vi "Teleop.vi"(10 "Match Info":T2={"Autonomous Elapsed Seconds"=0.0, "TeleOp Elapsed Seconds"=1423.678, "Disabled Elapsed Seconds"=30.39, "Visited Autonomous"=FALSE, "Visited TeleOp"=TRUE, "Visited Disabled"=TRUE, "Autonomous Settings"={"Autonomous Style"=enum."Independent", "VI Refnum"=refnum}}, 11 "Call Context":T3=enum."Execute") -> ()   [LabVIEW 2012]
doc: "This VI is called for each TeleOp packet received from the DS where the robot is not disabled. It is often used to read from the joysticks and update I/O or to update setpoints for timed control loops. It should complete and return within 20 milliseconds or it may miss DS packets."
uses:
  <vilib>/Rock Robotics/WPI/DriverStation/WPI_DriverStationDerivedRobotMode.ctl
  <vilib>/Rock Robotics/WPI/DriverStation/WPI_DriverStationMatch Info.ctl
  Driver/ADXL345 I2C Axis.ctl
  Robot Global Data.vi
  <vilib>/Rock Robotics/WPI/Solenoid/Deprecated/WPI_SolenoidSetBool.vi
  <vilib>/Rock Robotics/WPI/Joystick/WPI_JoystickGetSetRefNum.vi
panel:
  in  "Speed\nLoop Gain":dbl=1.5 step=0.1
  out "Speed feet/sec":dbl[](array[numeric])=[3.755830108947835e-15, 1.6772788571212362e-15] format="%#_4f"
  in  "Right Motor Speed":dbl(slide)=0.20408163265306145 scale=-10.0..10.0
  in  "Reset Gyro":bool
  in  "Reset Distance":bool
  out "Gyro\nAngle":dbl=356.1354393216929
  in  "SLGain\nOLD ROBOT":dbl=4.000000000000003 step=0.1
  out "Loop Time":dbl=0.023
  in  "Enable Speed Control":bool=TRUE
  out "Motor Chart":T1(graph)={"Right Motor Output"=-0.0009300018600037199, "Speed"=3.755830108947835e-15, "Speed"=1.6772788571212362e-15}
  out "Distance":dbl[](array[numeric])=[109.47032085561497, 100.94278074866311] format="%#_4f"
  out "Accelerometer Chart":cluster{"Output":dbl, dbl}(graph)={"Output"=-1.6895785716878318, -1.90123646461443}
  in  "Pitch avg.#":dbl=0.95
  out "Pitch Angle":dbl(knob)=-1.6895785716878318 scale=20.0..-20.0 scale format="%#_3g"
  in  "Left Motor Speed":dbl(slide)=0.4081632653061227 scale=-10.0..10.0
  in  "Enable Auto-Balance":bool
  out "Wheel Angles":dbl[](array[knob])=[15.270320855614973, 6.742780748663112] scale=0.0..18.84
  # "Speed Loop"
  # "1.5"
  # "4.0 on 2011 robot"
  # "2.5 on home unit"
  # "FOR TESTING ONLY"
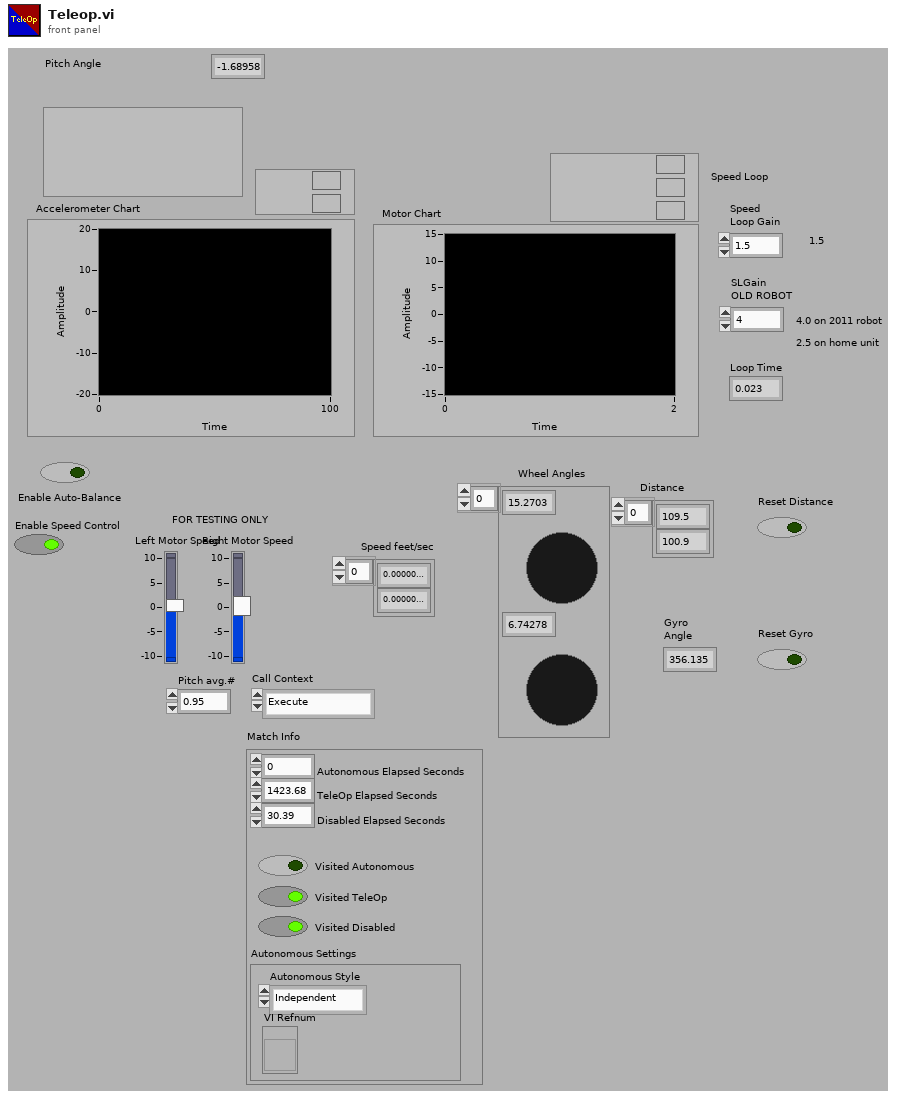
[diagram p1: front panel]
types:
  T1 = cluster{"Right Motor Output":dbl, "Speed":dbl, "Speed":dbl}
  T2 = typedef "WPI_DriverStationMatch Info.ctl" = cluster{"Autonomous Elapsed Seconds":dbl, "TeleOp Elapsed Seconds":dbl, "Disabled Elapsed Seconds":dbl, "Visited Autonomous":bool, "Visited TeleOp":bool, "Visited Disabled":bool, "Autonomous Settings":cluster{"Autonomous Style":enum16{"Iterative", "Independent"}, "VI Refnum":refnum<vi>}}
  T3 = typedef "WPI_DriverStationDerivedRobotMode.ctl" = enum16{"Init", "Execute", "Stop"}
  T4 = typedef "ADXL345 I2C Axis.ctl" = u8
  T5 = typedef "WPI_JoystickDevRef.ctl" = cluster{"Device":T6}
  T6 = typedef "WPI_JoystickDeviceEnum.ctl" = enum16{"USB 1", "USB 2", "USB 3", "USB 4", "Kinect 1", "Kinect 2"}
  T7 = typedef "WPI_JoystickButtonState.ctl" = cluster{"Button 1":bool, "Button 2":bool, "Button 3":bool, "Button 4":bool, "Button 5":bool, "Button 6":bool, "Button 7":bool, "Button 8":bool, "Button 9":bool, "Button 10":bool, "Button 11":bool, "Button 12":bool}
  T8 = typedef "WPI_SolenoidDevRef.ctl" = cluster{"DevStatus":errorcluster, "Solenoid Module":T9, "Forward Solenoid Channel":T10, "Reverse Solenoid Channel":T10}
  T9 = typedef "FPGA_TypedefSolenoidModule.ctl" = enum16{"Solenoid Module 1", "Solenoid Module 2"}
  T10 = typedef "WPI_SolenoidChannel.ctl" = enum8{"Solenoid 1", "Solenoid 2", "Solenoid 3", "Solenoid 4", "Solenoid 5", "Solenoid 6", "Solenoid 7", "Solenoid 8", "Invalid"}
  T11 = typedef "WPI_I2CDevRef.ctl" = cluster{"DevStatus":errorcluster, "Digital Module":T12, "Device Address":u8}
  T12 = typedef "FPGA_TypedefDigitalModule.ctl" = enum16{"Digital Module 1", "Digital Module 2"}
  T13 = cluster{"Left Motor Out":dbl, "Current angle (deg)":dbl, "Current angle (deg)":dbl}
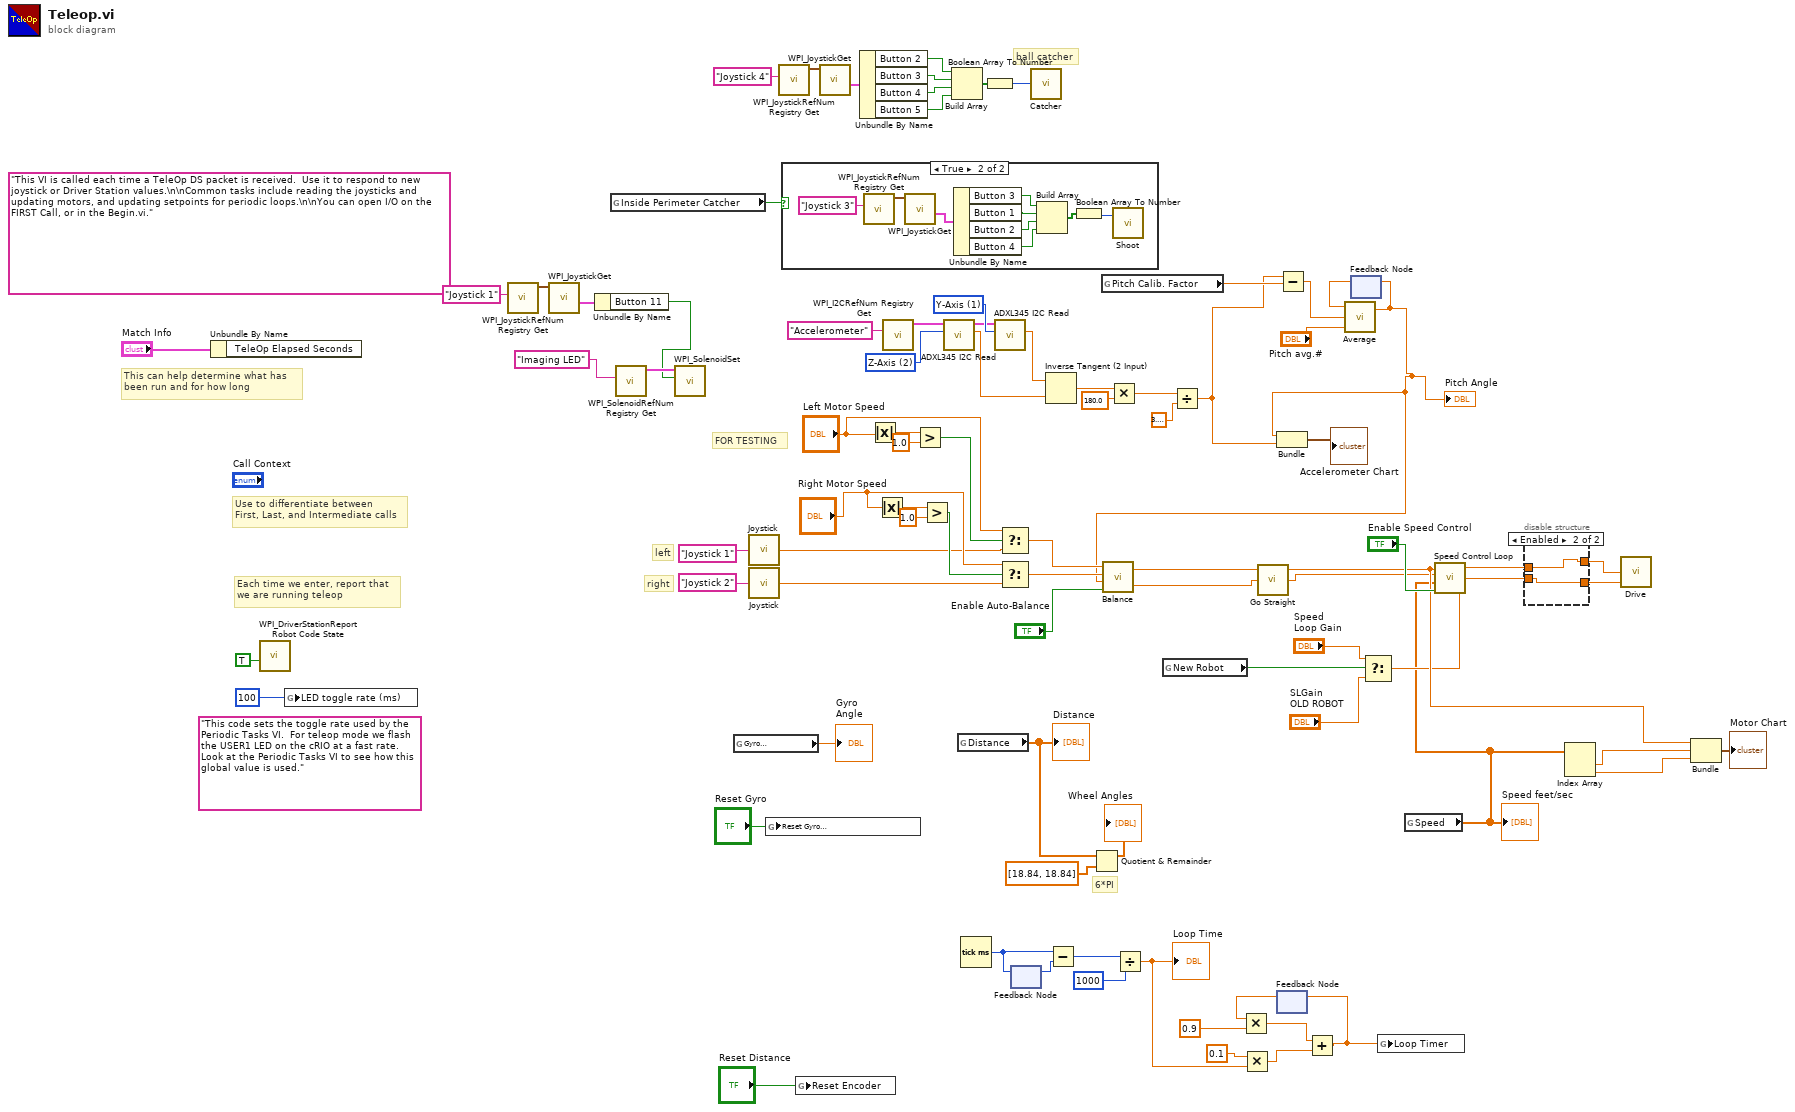
[diagram p0: block diagram]
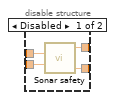
[diagram p2: hidden frame]
diagram:
  w40 = T4 2 items=["X-Axis", "Y-Axis", "Z-Axis"] ("Axis")
  w41 = T4 1 items=["X-Axis", "Y-Axis", "Z-Axis"] ("Axis")
  (unwired) "This code sets the toggle rate used by the Periodic Tasks VI.  For teleop mode we flash the USER1 LED on the cRIO at a fast rate.  Look at the Periodic Tasks VI to see how this global value is used."
  (unwired) "This VI is called each time a TeleOp DS packet is received.  Use it to respond to new joystick or Driver Station values.\n\nCommon tasks include reading the joysticks and updating motors, and updating setpoints for periodic loops.\n\nYou can open I/O on the FIRST Call, or in the Begin.vi."
  # "ball catcher"
  # "6*PI"
  # "FOR TESTING"
  # "right"
  # "left"
  # "Each time we enter, report that\nwe are running teleop"
  # "Use to differentiate between\nFirst, Last, and Intermediate calls"
  # "This can help determine what has\nbeen run and for how long"
  n1 = Unbundle By Name("Match Info") -> ()  [unwired: 1 out]
  n2 = call <vilib>:"WPI_DriverStationReport Robot Code State.vi"("TeleOp"=TRUE ("Autonomous")) -> ()  [unwired: 10 in, 1 out]
  n3 = global write "Robot Global Data.vi" "LED toggle rate (ms)"(u32 100 ("LED ms toggle rate")) -> ()
  n4 = call <vilib>:"WPI_JoystickRefNum Registry Get.vi"("refnum name"="Joystick 1") -> ("JoystickDevRef"=w14:T5)  [unwired: 9 in, 1 out]
  n5 = call <vilib>:"WPI_JoystickGet.vi"("JoystickDevRef"=w14) -> ("Buttons"=w13:T7)  [unwired: 4 in, 2 out]
  n6 = Unbundle By Name(w13) -> ("Button 11"=w10:bool)
  n7 = global read "Robot Global Data.vi" "Inside Perimeter Catcher"() -> (w19:bool)
  n8 = call <vilib>:"WPI_SolenoidRefNum Registry Get.vi"("refnum name"="Imaging LED") -> ("SolenoidDevRef"=w12:T8)  [unwired: 9 in, 1 out]
  n9 = call-poly <vilib>:"WPI_SolenoidSet.vi"("Value"=w10, "SolenoidDevRef"=w12) -> ()  [unwired: 8 in, 2 out]
  n10 = global read "Robot Global Data.vi" "Gyro\nAngle"() -> (→"Gyro\nAngle":dbl)
  n11 = call "Joystick.vi"("Joystick Refnum In"="Joystick 1" ("refnum name")) -> ("Speed Out"=w51:dbl)
  n12 = call "Joystick.vi"("Joystick Refnum In"="Joystick 2" ("refnum name")) -> ("Speed Out"=w50:dbl)
  n13 = global write "Robot Global Data.vi" "Reset Gyro\nZero Position"("Reset Gyro") -> ()
  n14 = call <vilib>:"WPI_JoystickRefNum Registry Get.vi"("refnum name"="Joystick 4") -> ("JoystickDevRef"=w8:T5)  [unwired: 9 in, 1 out]
  n15 = case shown="True" w19 {
    frame False {
    }
    frame True {
      n16 = call <vilib>:"WPI_JoystickRefNum Registry Get.vi"("refnum name"="Joystick 3") -> ("JoystickDevRef"=w94:T5)  [unwired: 9 in, 1 out]
      n17 = call <vilib>:"WPI_JoystickGet.vi"("JoystickDevRef"=w94) -> ("Buttons"=w91:T7)  [unwired: 4 in, 2 out]
      n18 = Unbundle By Name(w91) -> ("Button 3"=w93:bool, "Button 1"=w89:bool, "Button 2"=w88:bool, "Button 4"=w87:bool)
      n19 = Build Array(w93, w89, w88, w87) -> (w92:bool[])
      n20 = Boolean Array To Number(Boolean array=w92) -> (number=w90:u32)
      n21 = call "Shoot.vi"("Shooter Position (0 to 8)"=w90) -> ()  [unwired: 1 in, 2 out]
    }
  }
  n22 = global write "Robot Global Data.vi" "Reset Encoder"("Reset Distance") -> ()
  n23 = call <vilib>:"WPI_JoystickGet.vi"("JoystickDevRef"=w8) -> ("Buttons"=w7:T7)  [unwired: 4 in, 2 out]
  n24 = Unbundle By Name(w7) -> ("Button 2"=w3:bool, "Button 3"=w6:bool, "Button 4"=w5:bool, "Button 5"=w4:bool)
  n25 = Absolute Value(x="Left Motor Speed") -> (abs(x)=w76:dbl)
  n26 = Absolute Value(x="Right Motor Speed") -> (abs(x)=w55:dbl)
  n27 = call <vilib>:"WPI_I2CRefNum Registry Get.vi"("refnum name"="Accelerometer") -> ("I2CDevRef"=w37:T11)  [unwired: 9 in, 1 out]
  n28 = Greater?(x=w76, y=1.0) -> (0:w78:bool)
  n29 = Greater?(x=w55, y=1.0) -> (0:w53:bool)
  n30 = call "ADXL345 I2C Read.vi"("Axis"=w40, "I2CDevRef"=w37) -> ("Acceleration"=w43:dbl, "I2CDevRef Out"=w39:T11)  [unwired: 1 in, 7 out]
  n31 = Build Array(w3, w6, w5, w4) -> (w2:bool[])
  n32 = global read "Robot Global Data.vi" "Distance"() -> (w59:dbl[])
  "Distance" <- w59
  n33 = Tick Count (ms)() -> (millisecond timer value=w72:u32)
  n34 = Boolean Array To Number(Boolean array=w2) -> (number=w1:u32)
  n35 = call "ADXL345 I2C Read.vi"("Axis"=w41, "I2CDevRef"=w39) -> ("Acceleration"=w42:dbl)  [unwired: 1 in, 8 out]
  n36 = Select(t="Left Motor Speed", s=w78, f=w51) -> (s? t:f=w80:dbl)
  n37 = Select(t="Right Motor Speed", s=w53, f=w50) -> (s? t:f=w79:dbl)
  n38 = feedback #1() -> (w73:u32)  [unwired: 1 in]
  n39 = feedback-in #1(w72) -> ()
  n40 = call "Catcher.vi"("Catcher Position"=w1) -> ()
  n41 = Inverse Tangent (2 Input)(1:w43, 2:w42) -> (0:w44:dbl)
  n42 = Subtract(x=w72, y=w73) -> (x-y=w71:u32)
  n43 = Quotient & Remainder(x=w59, y=dbl[] [18.84, 18.84]) -> (x-y*floor(x/y)=→"Wheel Angles":dbl[])  [unwired: 1 out]
  n44 = global read "Robot Global Data.vi" "Pitch Calib. Factor"() -> (w22:dbl)
  n45 = Multiply(x=w44, y=180.0) -> (x*y=w66:dbl)
  n46 = Divide(x=w71, y=u32 1000) -> (x/y=w25:dbl)
  "Loop Time" <- w25
  n47 = global read "Robot Global Data.vi" "New Robot"() -> (w24:bool)
  n48 = Divide(x=w66, y=3.141592653589793) -> (x/y=w21:dbl)
  n49 = Multiply(x=0.1, y=w25) -> (x*y=w27:dbl)
  n50 = feedback #2() -> (w29:dbl)  [unwired: 1 in]
  n51 = Multiply(x=w29, y=0.9) -> (x*y=w28:dbl)
  n52 = Subtract(x=w21, y=w22) -> (x-y=w20:dbl)
  n53 = Add(x=w28, y=w27) -> (x+y=w31:dbl)
  n54 = feedback-in #2(w31) -> ()
  n55 = feedback #3() -> (w63:dbl)  [unwired: 1 in]
  n56 = call "Average.vi"("averg #"="Pitch avg.#", "Input"=w20, "Previous\nValue"=w63) -> ("Output"=w23:dbl)  [unwired: 1 in]
  "Pitch Angle" <- w23
  n57 = call "Balance.vi"("Balance Enabled"="Enable Auto-Balance", "Measured Angle"=w23, "Right Motor Input"=w79, "Left Motor Input"=w80) -> ("Right Motor Output"=w48:dbl, "Left Motor Output"=w49:dbl)
  n58 = call "Go Straight.vi"("Right Motor In"=w48, "Left Motor In"=w49) -> ("Right Motor Out"=w46:dbl, "Left Motor Out"=w47:dbl)  [unwired: 2 in]
  n59 = Bundle("Output"=w23, w21) -> (→"Accelerometer Chart":cluster{"Output":dbl, dbl})  [unwired: 1 in]
  n60 = feedback-in #3(w23) -> ()
  n61 = Select(t="Speed\nLoop Gain", s=w24, f="SLGain\nOLD ROBOT") -> (s? t:f=w36:dbl)
  n62 = global write "Robot Global Data.vi" "Loop Timer"(w31) -> ()
  n63 = global read "Robot Global Data.vi" "Speed"() -> (w16:dbl[])
  "Speed feet/sec" <- w16
  n64 = call "Speed Control Loop.vi"("Loop Gain"=w36, "Enable Speed Control"="Enable Speed Control", "Speed Feet/Minute"=w16, "Right Motor IN"=w46, "Left Motor IN"=w47) -> ("Right Motor OUT"=w33:dbl, "Left Motor OUT"=w32:dbl)
  n65 = disable-structure shown="Enabled" {
    disable-tunnel: w33 -> [w99 w100]
    disable-tunnel: w32 -> [w98 w101]
    disable-tunnel: [w97 w100] -> w18
    disable-tunnel: [w96 w101] -> w17
    frame Disabled {
      n66 = call "Sonar safety.vi"("M1 input"=w98, "M2 input"=w99) -> ("M1 Output"=w96:dbl, "M2 output"=w97:dbl)  [unwired: 1 in]
    }
    frame Enabled {
    }
  }
  n67 = Index Array(array=w16) -> (element #1=w75:dbl, element #2=w74:dbl)  [unwired: 2 in]
  n68 = call "Drive.vi"("Right Motor IN"=w18, "Left Motor IN"=w17) -> ()  [unwired: 3 in, 1 out]
  n69 = Bundle("Left Motor Out"=w47, "Current angle (deg)"=w75, "Current angle (deg)"=w74) -> (→"Motor Chart":T13)  [unwired: 1 in]
